vi "Find First Tag.vi"(11 "XML String":string) -> (0 "Attributes":map{string, string}(c390), 1 "Data":string, 2 "Tag Name":string, 3 "XML After First Tag":string, 4 "Flags":T1)   [LabVIEW 2021, in "Tree Map.lvlib"]
doc: "<b>Author:</b> Piotr Kruczkowski <PrimaryKey>\n<b>License:</b> NewBSD\n\nCopyright (c) 2019, National Instruments\nAll rights reserved.\n\nRedistribution and use in source and binary forms, with or without\nmodification, are permitted provided that the following conditions are met:\n1. Redistributions of source code must retain the above copyright\n notice, this list of conditions and the following disclaimer.\n2. Redistributions in binary form must reproduce the above copyright\n notice, this list of conditions and the following disclaimer in the\n documentation and/or other materials provided with the distribution.\n3. Neither the name of National Instruments nor the\n names of its contributors may be used to endorse or promote products\n derived from this software without specific prior written permission.\n\nTHIS SOFTWARE IS PROVIDED BY National Instruments ''AS IS'' AND ANY\nEXPRESS OR IMPLIED WARRANTIES, INCLUDING, BUT NOT LIMITED TO, THE IMPLIED\nWARRANTIES OF MERCHANTABILITY AND FITNESS FOR A PARTICULAR PURPOSE ARE\nDISCLAIMED. IN NO EVENT SHALL National Instruments BE LIABLE FOR ANY\nDIRECT, INDIRECT, INCIDENTAL, SPECIAL, EXEMPLARY, OR CONSEQUENTIAL DAMAGES\n(INCLUDING, BUT NOT LIMITED TO, PROCUREMENT OF SUBSTITUTE GOODS OR SERVICES;\nLOSS OF USE, DATA, OR PROFITS; OR BUSINESS INTERRUPTION) HOWEVER CAUSED AND\nON ANY THEORY OF LIABILITY, WHETHER IN CONTRACT, STRICT LIABILITY, OR TORT\n(INCLUDING NEGLIGENCE OR OTHERWISE) ARISING IN ANY WAY OUT OF THE USE OF THIS\nSOFTWARE, EVEN IF ADVISED OF THE POSSIBILITY OF SUCH DAMAGE."
uses:
  <vilib>/National Instruments/Tree Map/Tree Map.lvlib
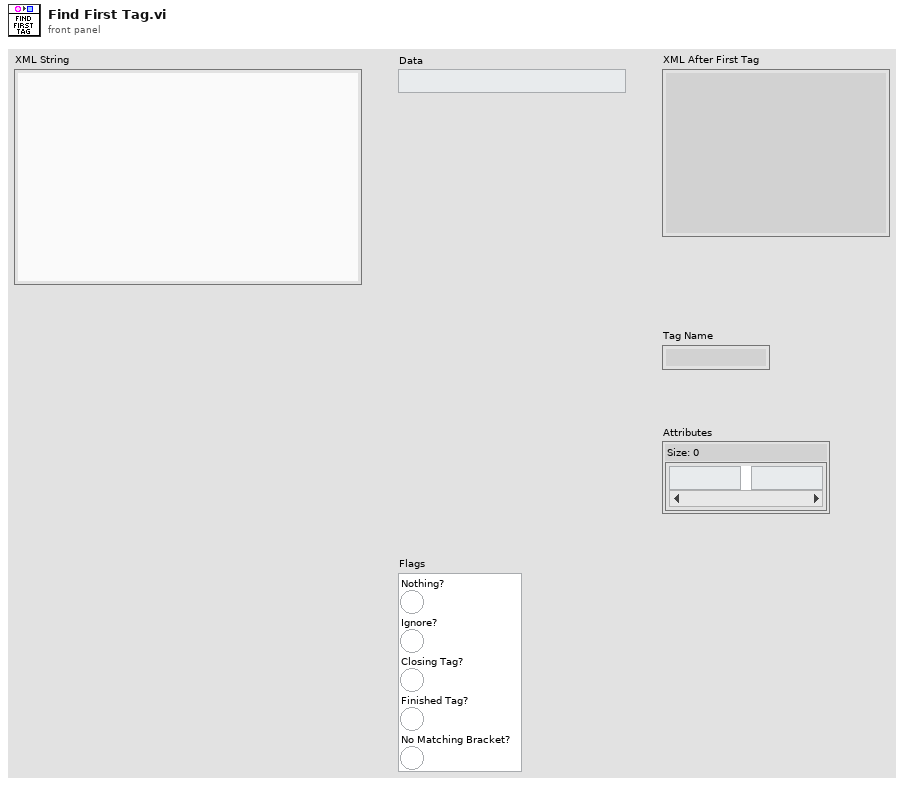
[diagram p1: front panel]
types:
  T1 = cluster{"Nothing?":bool, "Ignore?":bool, "Closing Tag?":bool, "Finished Tag?":bool, "No Matching Bracket?":bool}
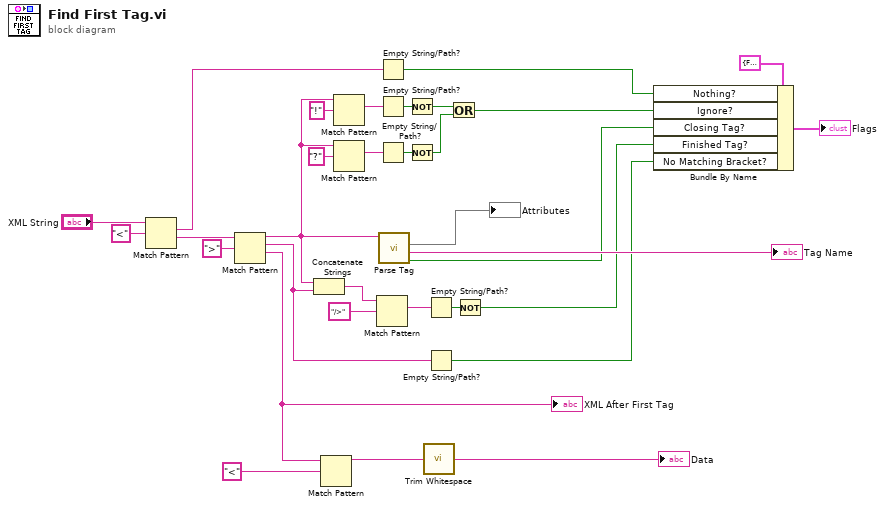
[diagram p0: block diagram]
diagram:
  n1 = Match Pattern(string="XML String", regular expression="<") -> (match substring=w30:string, after substring=w18:string)  [unwired: 1 in, 2 out]
  n2 = Match Pattern(string=w18, regular expression=">") -> (before substring=w14:string, match substring=w26:string, after substring=w3:string)  [unwired: 1 in, 1 out]
  "XML After First Tag" <- w3
  n3 = Concatenate Strings(w14, w26) -> (w25:string)
  n4 = Match Pattern(string=w3, regular expression="<") -> (before substring=w2:string)  [unwired: 1 in, 3 out]
  n5 = Match Pattern(string=w14, regular expression="!") -> (match substring=w20:string)  [unwired: 1 in, 3 out]
  n6 = Match Pattern(string=w14, regular expression="?") -> (match substring=w23:string)  [unwired: 1 in, 3 out]
  n7 = Match Pattern(string=w25, regular expression="/>") -> (match substring=w28:string)  [unwired: 1 in, 3 out]
  n8 = Empty String/Path?(string/path=w30) -> (empty?=w10:bool)
  n9 = Empty String/Path?(string/path=w20) -> (empty?=w21:bool)
  n10 = Empty String/Path?(string/path=w23) -> (empty?=w22:bool)
  n11 = call <vilib>:"Parse Tag.vi"("Tag String"=w14) -> ("</ Tag>"=w8:bool, "Tag Name"=→"Tag Name":string, "Attributes"=→"Attributes":map{string, string})  [unwired: 8 in]
  n12 = Not(x=w21) -> (.not. x?=w16:bool)
  n13 = Not(x=w22) -> (.not. x?=w17:bool)
  n14 = call <vilib>:"Trim Whitespace.vi"("string"=w2) -> ("trimmed string"=→"Data":string)  [unwired: 1 in]
  n15 = Empty String/Path?(string/path=w28) -> (empty?=w27:bool)
  n16 = Empty String/Path?(string/path=w26) -> (empty?=w6:bool)
  n17 = Or(x=w16, y=w17) -> (x .or. y?=w9:bool)
  n18 = Not(x=w27) -> (.not. x?=w7:bool)
  n19 = Bundle By Name(cluster=T1 {"Nothing?"=FALSE, "Ignore?"=FALSE, "Closing Tag?"=FALSE, "Finished Tag?"=FALSE, "No Matching Bracket?"=FALSE} ("Flags"), "Nothing?"=w10, "Ignore?"=w9, "Closing Tag?"=w8, "Finished Tag?"=w7, "No Matching Bracket?"=w6) -> (→"Flags":T1)
